vi "CalculateBMonly.vi"() -> ()   [LabVIEW 2016]
uses:
  <vilib>/Utility/file.llb/Read Delimited Spreadsheet (string).vi
panel:
  in  "nm/pixel":dbl
  out "size(s) 2":i32
  out "Array":dbl[](array[numeric])
  out "size(s)":i32
  in  "±":dbl
  in  "BM":dbl
  out "BM lower limit":dbl
  out "BM upper limit":dbl
  in  "r should less than":dbl
  in  "x/y lower limit":dbl
  in  "x/y upper limit":dbl
  in  "BM range":bool
  in  "Relation coefficient":bool
  in  "rotate?":bool
  in  "x/y":bool
  out "all y position\n(pixel)":dbl[][](array[numeric])
  out "all x position\n(pixel)":dbl[][](array[numeric])
  out "# of frames":dbl
  out "# of AOIs":dbl
  out "Tandem Yi position":dbl[](array[numeric])
  out "Tandem Xi position":dbl[](array[numeric])
  out "Filenames":string[](array[string])
  out "path out":path
  in  "Path Folder":path
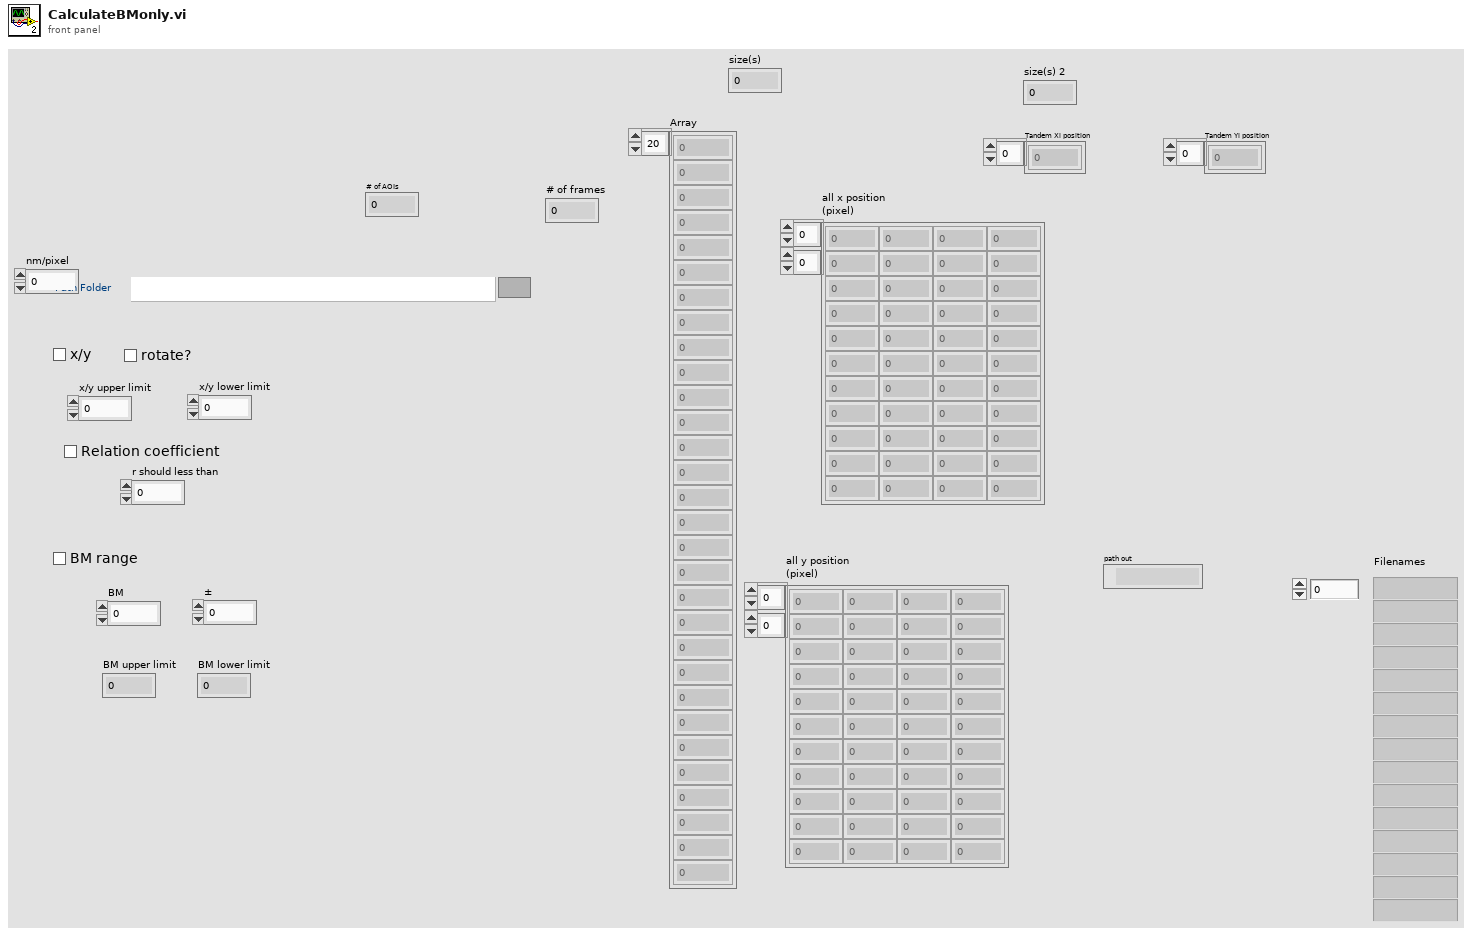
[diagram p1: front panel]
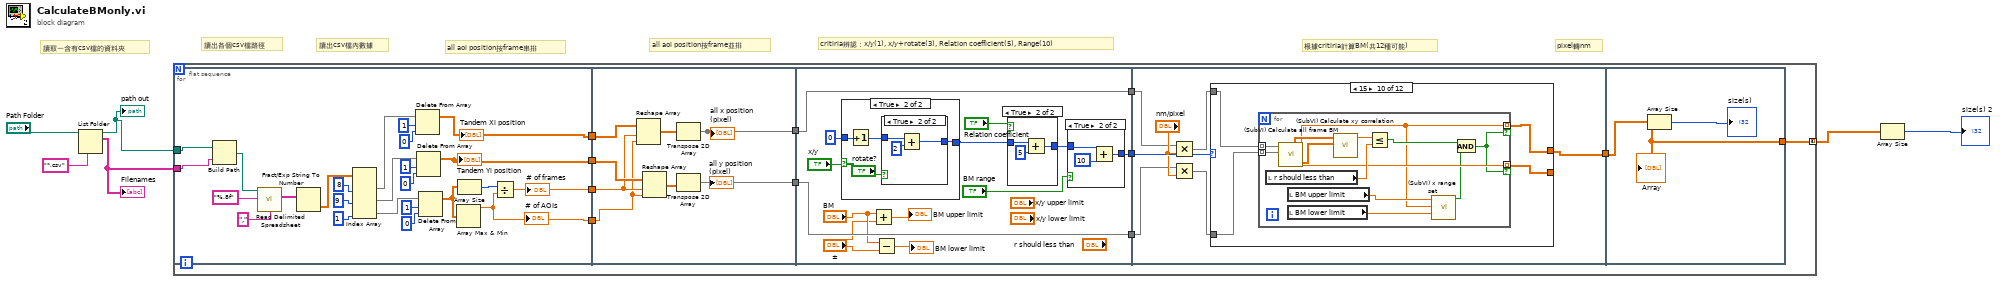
[diagram p0: block diagram]
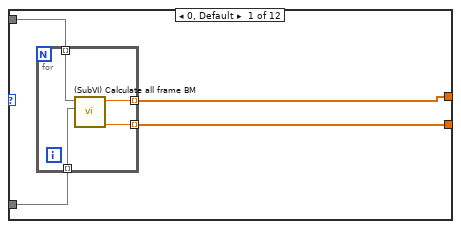
[diagram p6: hidden frame]
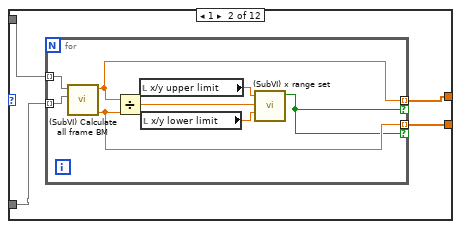
[diagram p7: hidden frame]
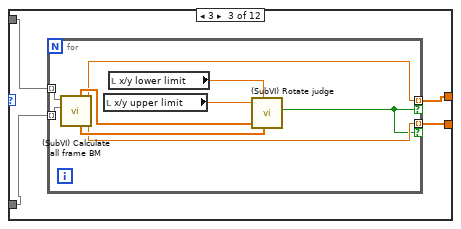
[diagram p8: hidden frame]
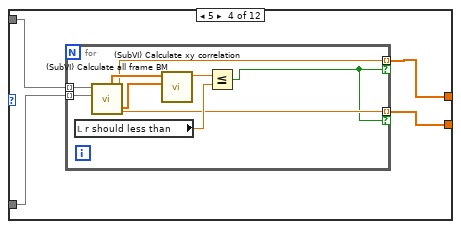
[diagram p9: hidden frame]
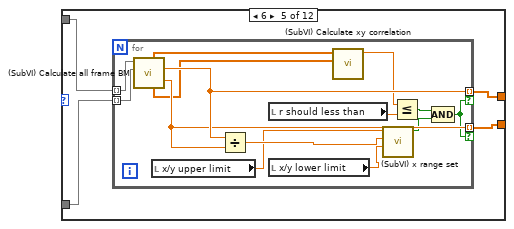
[diagram p10: hidden frame]
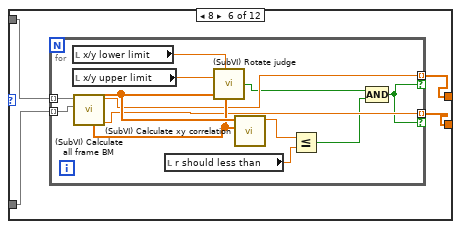
[diagram p11: hidden frame]
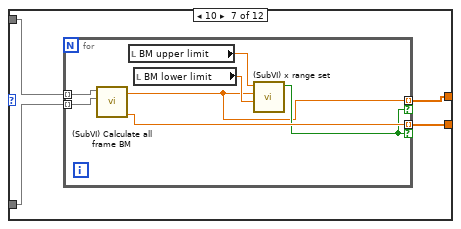
[diagram p12: hidden frame]
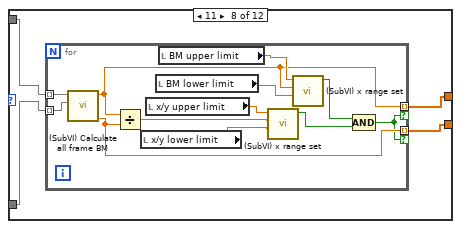
[diagram p13: hidden frame]
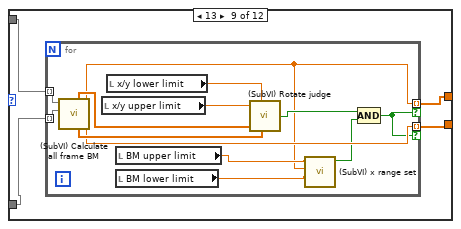
[diagram p14: hidden frame]
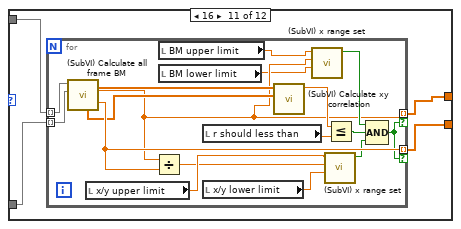
[diagram p15: hidden frame]
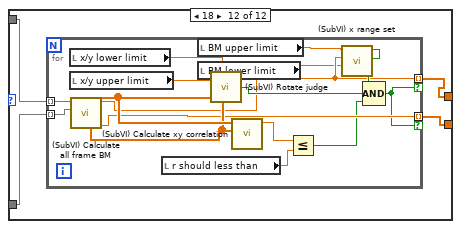
[diagram p16: hidden frame]
diagram:
  # "pixel轉nm"
  # "根據critiria計算BM(共12種可能)"
  # "critiria辨認：x/y(1), x/y+rotate(3), Relation coefficient(5), Range(10)"
  # "all aoi position按frame並排"
  # "all aoi position按frame串排"
  # "讀出csv檔內數據"
  # "讀出各個csv檔路徑"
  # "讀取一含有csv檔的資料夾"
  n1 = List Folder(path="Path Folder", pattern="*.csv") -> (path out=w4:path, filenames=w3:string[])  [unwired: 2 in, 2 out]
  "Filenames" <- w3
  "path out" <- w4
  n2 = for {
    tunnel: w4 -> [w9]
    tunnel: w3 -> [w8] mode=indexing
    tunnel: [w7] -> w1 mode=concatenating
    n3 = flat-sequence {
      tunnel: [w44] -> w19
      tunnel: [w43] -> w18
      tunnel: [w42] -> w17
      tunnel: [w41] -> w16
      tunnel: w9 -> [w40]
      tunnel: w8 -> [w39]
      tunnel: w19 -> [w52]
      tunnel: w18 -> [w51]
      tunnel: w17 -> [w50]
      tunnel: w16 -> [w49]
      tunnel: [w48] -> w15
      tunnel: [w47] -> w14
      tunnel: w15 -> [w58]
      tunnel: w14 -> [w57]
      tunnel: [w59] -> w13
      tunnel: [w58] -> w12
      tunnel: [w57] -> w11
      tunnel: w13 -> [w89]
      tunnel: w12 -> [w86]
      tunnel: w11 -> [w84]
      tunnel: [w87] -> w10
      tunnel: w10 -> [w273]
      tunnel: [w273] -> w7
      frame #0 {
        n4 = Build Path(base path=w40, name or relative path=w39) -> (appended path=w38:path)
        n5 = call-poly <vilib>:"Read Delimited Spreadsheet.vi"("file path (dialog if empty)"=w38, "format (%s)"="%.8f", "delimiter (\\t)"="," ("delimiter (\\t)")) -> ("all rows"=w35:string[][])  [unwired: 7 in, 5 out]
        n6 = Fract/Exp String To Number(string=w35) -> (number=w34:dbl[][])  [unwired: 3 in, 1 out]
        n7 = Index Array(array=w34, index (col) #1=8 ("disabled index (col)"), index (col) #2=9 ("index (col)"), index (col) #3=1 ("index (col)")) -> (element #1=w24:dbl[], element #2=w23:dbl[], element #3=w22:dbl[])  [unwired: 3 in]
        n8 = Delete From Array(array=w24, length=1, index=0) -> (array with subset deleted=w44:dbl[])  [unwired: 1 out]
        "Tandem Xi position" <- w44
        n9 = Delete From Array(array=w23, length=1, index=0) -> (array with subset deleted=w43:dbl[])  [unwired: 1 out]
        "Tandem Yi position" <- w43
        n10 = Delete From Array(array=w22, length=1, index=0) -> (array with subset deleted=w21:dbl[])  [unwired: 1 out]
        n11 = Array Max & Min(array=w21) -> (max value=w41:dbl)  [unwired: 3 out]
        "# of AOIs" <- w41
        n12 = Array Size(array=w21) -> (size(s)=w20:i32)
        n13 = Divide(x=w20, y=w41) -> (x/y=w42:dbl)
        "# of frames" <- w42
      }
      frame #1 {
        n14 = Reshape Array(w52, w50, w49) -> (w46:dbl[][])
        n15 = Reshape Array(w51, w50, w49) -> (w45:dbl[][])
        n16 = Transpose 2D Array(2D array=w45) -> (transposed array=w47:dbl[][])
        "all y position\n(pixel)" <- w47
        n17 = Transpose 2D Array(2D array=w46) -> (transposed array=w48:dbl[][])
        "all x position\n(pixel)" <- w48
      }
      frame #2 {
        n18 = case shown="True" "x/y" {
          tunnel: 0 -> [w74 w78]
          tunnel: [w74 w75] -> w62
          frame False {
          }
          frame True {
            n19 = Increment(x=w78) -> (x+1=w76:i32)
            n20 = case shown="True" "rotate?" {
              tunnel: w76 -> [w79 w81]
              tunnel: [w79 w80] -> w75
              frame False {
              }
              frame True {
                n21 = Add(x=w81, y=2) -> (x+y=w80:i32)
              }
            }
          }
        }
        n22 = Add(x="BM", y="±") -> (x+y=→"BM upper limit":dbl)
        n23 = Subtract(x="BM", y="±") -> (x-y=→"BM lower limit":dbl)
        n24 = case shown="True" "Relation coefficient" {
          tunnel: w62 -> [w70 w72]
          tunnel: [w70 w71] -> w65
          frame False {
          }
          frame True {
            n25 = Add(x=w72, y=5) -> (x+y=w71:i32)
          }
        }
        n26 = case shown="True" "BM range" {
          tunnel: w65 -> [w66 w68]
          tunnel: [w66 w67] -> w59
          frame False {
          }
          frame True {
            n27 = Add(x=w68, y=10) -> (x+y=w67:i32)
          }
        }
      }
      frame #3 {
        n28 = Multiply(x=w86, y="nm/pixel") -> (x*y=w85:dbl[][])
        n29 = Multiply(x=w84, y="nm/pixel") -> (x*y=w83:dbl[][])
        n30 = case shown="15" w89 {
          tunnel: w85 -> [w93 w101 w113 w126 w139 w157 w174 w185 w201 w218 w235 w256]
          tunnel: w83 -> [w92 w100 w112 w125 w138 w156 w173 w184 w200 w217 w234 w255]
          tunnel: [w91 w99 w111 w124 w137 w155 w172 w183 w199 w216 w233 w254] -> w87
          tunnel: [w90 w98 w110 w123 w136 w154 w171 w182 w198 w215 w232 w253] -> _
          frame 0, Default {
            n31 = for {
              tunnel: w93 -> [w97] mode=indexing
              tunnel: w92 -> [w96] mode=indexing
              tunnel: [w95] -> w91 mode=indexing
              tunnel: [w94] -> w90 mode=indexing
              n32 = call "(SubVI) Calculate all frame BM.vi"("y position (pixel)"=w96, "x position (pixel)"=w97) -> ("y standard deviation"=w94:dbl, "x standard deviation"=w95:dbl)  [unwired: 6 in, 2 out]
            }
          }
          frame 1 {
            n33 = for {
              tunnel: [w109] -> w99 mode=indexing if=w102
              tunnel: [w108] -> w98 mode=indexing if=w102
              tunnel: w101 -> [w107] mode=indexing
              tunnel: w100 -> [w106] mode=indexing
              n34 = call "(SubVI) Calculate all frame BM.vi"("y position (pixel)"=w106, "x position (pixel)"=w107) -> ("y standard deviation"=w108:dbl, "x standard deviation"=w109:dbl)  [unwired: 6 in, 2 out]
              n35 = Divide(x=w109, y=w108) -> (x/y=w104:dbl)
              n36 = local read "x/y upper limit"() -> (w105:dbl)
              n37 = local read "x/y lower limit"() -> (w103:dbl)
              n38 = call "(SubVI) x range set.vi"("lower limit"=w103, "x"=w104, "upper limit"=w105) -> ("Boolean"=w102:bool)  [unwired: 8 in]
            }
          }
          frame 3 {
            n39 = for {
              tunnel: w113 -> [w122] mode=indexing
              tunnel: w112 -> [w121] mode=indexing
              tunnel: [w116] -> w111 mode=indexing if=w114
              tunnel: [w115] -> w110 mode=indexing if=w114
              n40 = call "(SubVI) Calculate all frame BM.vi"("y position (pixel)"=w121, "x position (pixel)"=w122) -> ("y standard deviation"=w115:dbl, "x standard deviation"=w116:dbl, "y position (delete y fit error)"=w119:dbl[], "x position (delete x fit error)"=w120:dbl[])  [unwired: 6 in]
              n41 = local read "x/y upper limit"() -> (w118:dbl)
              n42 = local read "x/y lower limit"() -> (w117:dbl)
              n43 = call "(SubVI) Rotate judge.vi"("x/y upper limit"=w118, "x/y lower limit"=w117, "x position (delete y fit error)"=w120, "y position (delete y fit error)"=w119) -> ("x = y?"=w114:bool)  [unwired: 1 in]
            }
          }
          frame 5 {
            n44 = for {
              tunnel: w126 -> [w135] mode=indexing
              tunnel: w125 -> [w134] mode=indexing
              tunnel: [w129] -> w124 mode=indexing if=w127
              tunnel: [w128] -> w123 mode=indexing if=w127
              n45 = local read "r should less than"() -> (w130:dbl)
              n46 = call "(SubVI) Calculate all frame BM.vi"("y position (pixel)"=w134, "x position (pixel)"=w135) -> ("y standard deviation"=w128:dbl, "x standard deviation"=w129:dbl, "y position (delete y fit error)"=w132:dbl[], "x position (delete x fit error)"=w133:dbl[])  [unwired: 6 in]
              n47 = call "(SubVI) Calculate xy correlation.vi"("y position (delete y fit error)"=w132, "x position (delete x fit error)"=w133) -> ("Numeric"=w131:dbl)  [unwired: 9 in]
              n48 = Less Or Equal?(x=w131, y=w130) -> (x <= y?=w127:bool)
            }
          }
          frame 6 {
            n49 = for {
              tunnel: w139 -> [w153] mode=indexing
              tunnel: w138 -> [w152] mode=indexing
              tunnel: [w151] -> w137 mode=indexing if=w145
              tunnel: [w150] -> w136 mode=indexing if=w145
              n50 = call "(SubVI) Calculate all frame BM.vi"("y position (pixel)"=w152, "x position (pixel)"=w153) -> ("y standard deviation"=w150:dbl, "x standard deviation"=w151:dbl, "y position (delete y fit error)"=w146:dbl[], "x position (delete x fit error)"=w147:dbl[])  [unwired: 6 in]
              n51 = local read "x/y upper limit"() -> (w141:dbl)
              n52 = Divide(x=w151, y=w150) -> (x/y=w142:dbl)
              n53 = local read "r should less than"() -> (w148:dbl)
              n54 = local read "x/y lower limit"() -> (w140:dbl)
              n55 = call "(SubVI) Calculate xy correlation.vi"("y position (delete y fit error)"=w146, "x position (delete x fit error)"=w147) -> ("Numeric"=w149:dbl)  [unwired: 9 in]
              n56 = call "(SubVI) x range set.vi"("lower limit"=w140, "x"=w142, "upper limit"=w141) -> ("Boolean"=w144:bool)  [unwired: 8 in]
              n57 = Less Or Equal?(x=w149, y=w148) -> (x <= y?=w143:bool)
              n58 = Compound Arithmetic op=AND(w143, w144) -> (w145:bool)
            }
          }
          frame 8 {
            n59 = for {
              tunnel: w157 -> [w170] mode=indexing
              tunnel: w156 -> [w169] mode=indexing
              tunnel: [w162] -> w155 mode=indexing if=w158
              tunnel: [w161] -> w154 mode=indexing if=w158
              n60 = local read "x/y lower limit"() -> (w165:dbl)
              n61 = local read "x/y upper limit"() -> (w166:dbl)
              n62 = call "(SubVI) Calculate all frame BM.vi"("y position (pixel)"=w169, "x position (pixel)"=w170) -> ("y standard deviation"=w161:dbl, "x standard deviation"=w162:dbl, "y position (delete y fit error)"=w167:dbl[], "x position (delete x fit error)"=w168:dbl[])  [unwired: 6 in]
              n63 = local read "r should less than"() -> (w163:dbl)
              n64 = call "(SubVI) Rotate judge.vi"("x/y upper limit"=w166, "x/y lower limit"=w165, "x position (delete y fit error)"=w168, "y position (delete y fit error)"=w167) -> ("x = y?"=w160:bool)  [unwired: 1 in]
              n65 = call "(SubVI) Calculate xy correlation.vi"("y position (delete y fit error)"=w167, "x position (delete x fit error)"=w168) -> ("Numeric"=w164:dbl)  [unwired: 9 in]
              n66 = Less Or Equal?(x=w164, y=w163) -> (x <= y?=w159:bool)
              n67 = Compound Arithmetic op=AND(w160, w159) -> (w158:bool)
            }
          }
          frame 10 {
            n68 = for {
              tunnel: w174 -> [w181] mode=indexing
              tunnel: w173 -> [w180] mode=indexing
              tunnel: [w175] -> w172 mode=indexing if=w178
              tunnel: [w179] -> w171 mode=indexing if=w178
              n69 = call "(SubVI) Calculate all frame BM.vi"("y position (pixel)"=w180, "x position (pixel)"=w181) -> ("y standard deviation"=w179:dbl, "x standard deviation"=w175:dbl)  [unwired: 6 in, 2 out]
              n70 = local read "BM upper limit"() -> (w177:dbl)
              n71 = local read "BM lower limit"() -> (w176:dbl)
              n72 = call "(SubVI) x range set.vi"("lower limit"=w176, "x"=w175, "upper limit"=w177) -> ("Boolean"=w178:bool)  [unwired: 8 in]
            }
          }
          frame 11 {
            n73 = for {
              tunnel: w185 -> [w197] mode=indexing
              tunnel: w184 -> [w196] mode=indexing
              tunnel: [w191] -> w183 mode=indexing if=w194
              tunnel: [w195] -> w182 mode=indexing if=w194
              n74 = call "(SubVI) Calculate all frame BM.vi"("y position (pixel)"=w196, "x position (pixel)"=w197) -> ("y standard deviation"=w195:dbl, "x standard deviation"=w191:dbl)  [unwired: 6 in, 2 out]
              n75 = Divide(x=w191, y=w195) -> (x/y=w187:dbl)
              n76 = local read "x/y lower limit"() -> (w186:dbl)
              n77 = local read "x/y upper limit"() -> (w189:dbl)
              n78 = local read "BM lower limit"() -> (w190:dbl)
              n79 = local read "BM upper limit"() -> (w192:dbl)
              n80 = call "(SubVI) x range set.vi"("lower limit"=w186, "x"=w187, "upper limit"=w189) -> ("Boolean"=w188:bool)  [unwired: 8 in]
              n81 = call "(SubVI) x range set.vi"("lower limit"=w190, "x"=w191, "upper limit"=w192) -> ("Boolean"=w193:bool)  [unwired: 8 in]
              n82 = Compound Arithmetic op=AND(w193, w188) -> (w194:bool)
            }
          }
          frame 13 {
            n83 = for {
              tunnel: w201 -> [w214] mode=indexing
              tunnel: w200 -> [w213] mode=indexing
              tunnel: [w203] -> w199 mode=indexing if=w206
              tunnel: [w208] -> w198 mode=indexing if=w206
              n84 = call "(SubVI) Calculate all frame BM.vi"("y position (pixel)"=w213, "x position (pixel)"=w214) -> ("y standard deviation"=w208:dbl, "x standard deviation"=w203:dbl, "y position (delete y fit error)"=w211:dbl[], "x position (delete x fit error)"=w212:dbl[])  [unwired: 6 in]
              n85 = local read "x/y upper limit"() -> (w210:dbl)
              n86 = local read "x/y lower limit"() -> (w209:dbl)
              n87 = local read "BM upper limit"() -> (w204:dbl)
              n88 = local read "BM lower limit"() -> (w202:dbl)
              n89 = call "(SubVI) Rotate judge.vi"("x/y upper limit"=w210, "x/y lower limit"=w209, "x position (delete y fit error)"=w212, "y position (delete y fit error)"=w211) -> ("x = y?"=w207:bool)  [unwired: 1 in]
              n90 = call "(SubVI) x range set.vi"("lower limit"=w202, "x"=w203, "upper limit"=w204) -> ("Boolean"=w205:bool)  [unwired: 8 in]
              n91 = Compound Arithmetic op=AND(w207, w205) -> (w206:bool)
            }
          }
          frame 15 {
            n92 = for {
              tunnel: w218 -> [w231] mode=indexing
              tunnel: w217 -> [w230] mode=indexing
              tunnel: [w220] -> w216 mode=indexing if=w223
              tunnel: [w225] -> w215 mode=indexing if=w223
              n93 = local read "r should less than"() -> (w226:dbl)
              n94 = call "(SubVI) Calculate all frame BM.vi"("y position (pixel)"=w230, "x position (pixel)"=w231) -> ("y standard deviation"=w225:dbl, "x standard deviation"=w220:dbl, "y position (delete y fit error)"=w228:dbl[], "x position (delete x fit error)"=w229:dbl[])  [unwired: 6 in]
              n95 = local read "BM upper limit"() -> (w221:dbl)
              n96 = local read "BM lower limit"() -> (w219:dbl)
              n97 = call "(SubVI) Calculate xy correlation.vi"("y position (delete y fit error)"=w228, "x position (delete x fit error)"=w229) -> ("Numeric"=w227:dbl)  [unwired: 9 in]
              n98 = Less Or Equal?(x=w227, y=w226) -> (x <= y?=w224:bool)
              n99 = call "(SubVI) x range set.vi"("lower limit"=w219, "x"=w220, "upper limit"=w221) -> ("Boolean"=w222:bool)  [unwired: 8 in]
              n100 = Compound Arithmetic op=AND(w224, w222) -> (w223:bool)
            }
          }
          frame 16 {
            n101 = for {
              tunnel: w235 -> [w252] mode=indexing
              tunnel: w234 -> [w251] mode=indexing
              tunnel: [w241] -> w233 mode=indexing if=w245
              tunnel: [w250] -> w232 mode=indexing if=w245
              n102 = call "(SubVI) Calculate all frame BM.vi"("y position (pixel)"=w251, "x position (pixel)"=w252) -> ("y standard deviation"=w250:dbl, "x standard deviation"=w241:dbl, "y position (delete y fit error)"=w246:dbl[], "x position (delete x fit error)"=w247:dbl[])  [unwired: 6 in]
              n103 = local read "x/y upper limit"() -> (w238:dbl)
              n104 = Divide(x=w241, y=w250) -> (x/y=w237:dbl)
              n105 = local read "BM upper limit"() -> (w242:dbl)
              n106 = local read "BM lower limit"() -> (w240:dbl)
              n107 = local read "r should less than"() -> (w248:dbl)
              n108 = local read "x/y lower limit"() -> (w236:dbl)
              n109 = call "(SubVI) Calculate xy correlation.vi"("y position (delete y fit error)"=w246, "x position (delete x fit error)"=w247) -> ("Numeric"=w249:dbl)  [unwired: 9 in]
              n110 = call "(SubVI) x range set.vi"("lower limit"=w240, "x"=w241, "upper limit"=w242) -> ("Boolean"=w243:bool)  [unwired: 8 in]
              n111 = call "(SubVI) x range set.vi"("lower limit"=w236, "x"=w237, "upper limit"=w238) -> ("Boolean"=w239:bool)  [unwired: 8 in]
              n112 = Less Or Equal?(x=w249, y=w248) -> (x <= y?=w244:bool)
              n113 = Compound Arithmetic op=AND(w243, w244, w239) -> (w245:bool)
            }
          }
          frame 18 {
            n114 = for {
              tunnel: w256 -> [w272] mode=indexing
              tunnel: w255 -> [w271] mode=indexing
              tunnel: [w258] -> w254 mode=indexing if=w261
              tunnel: [w264] -> w253 mode=indexing if=w261
              n115 = local read "x/y lower limit"() -> (w267:dbl)
              n116 = local read "x/y upper limit"() -> (w268:dbl)
              n117 = call "(SubVI) Calculate all frame BM.vi"("y position (pixel)"=w271, "x position (pixel)"=w272) -> ("y standard deviation"=w264:dbl, "x standard deviation"=w258:dbl, "y position (delete y fit error)"=w269:dbl[], "x position (delete x fit error)"=w270:dbl[])  [unwired: 6 in]
              n118 = local read "r should less than"() -> (w265:dbl)
              n119 = local read "BM upper limit"() -> (w259:dbl)
              n120 = local read "BM lower limit"() -> (w257:dbl)
              n121 = call "(SubVI) Rotate judge.vi"("x/y upper limit"=w268, "x/y lower limit"=w267, "x position (delete y fit error)"=w270, "y position (delete y fit error)"=w269) -> ("x = y?"=w263:bool)  [unwired: 1 in]
              n122 = call "(SubVI) Calculate xy correlation.vi"("y position (delete y fit error)"=w269, "x position (delete x fit error)"=w270) -> ("Numeric"=w266:dbl)  [unwired: 9 in]
              n123 = Less Or Equal?(x=w266, y=w265) -> (x <= y?=w262:bool)
              n124 = call "(SubVI) x range set.vi"("lower limit"=w257, "x"=w258, "upper limit"=w259) -> ("Boolean"=w260:bool)  [unwired: 8 in]
              n125 = Compound Arithmetic op=AND(w260, w263, w262) -> (w261:bool)
            }
          }
        }
      }
      frame #4 {
        n126 = Array Size(array=w273) -> (size(s)=→"size(s)":i32)
        "Array" <- w273
      }
    }
  }
  n127 = Array Size(array=w1) -> (size(s)=→"size(s) 2":i32)
